vi "Load WFM Data.vi"(4 "error in (no error)":errorcluster, 5 "# Records (1)":i32=1, 6 "# Records to Skip (0)":i32, 7 "Source File":path) -> (0 "error out":errorcluster, 3 "Data":waveform(dbl)[][](array[waveform]))   [LabVIEW 2013]
panel:
  out "Records read":i32
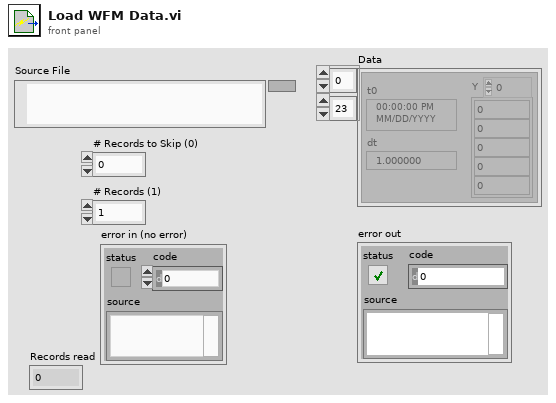
[diagram p1: front panel]
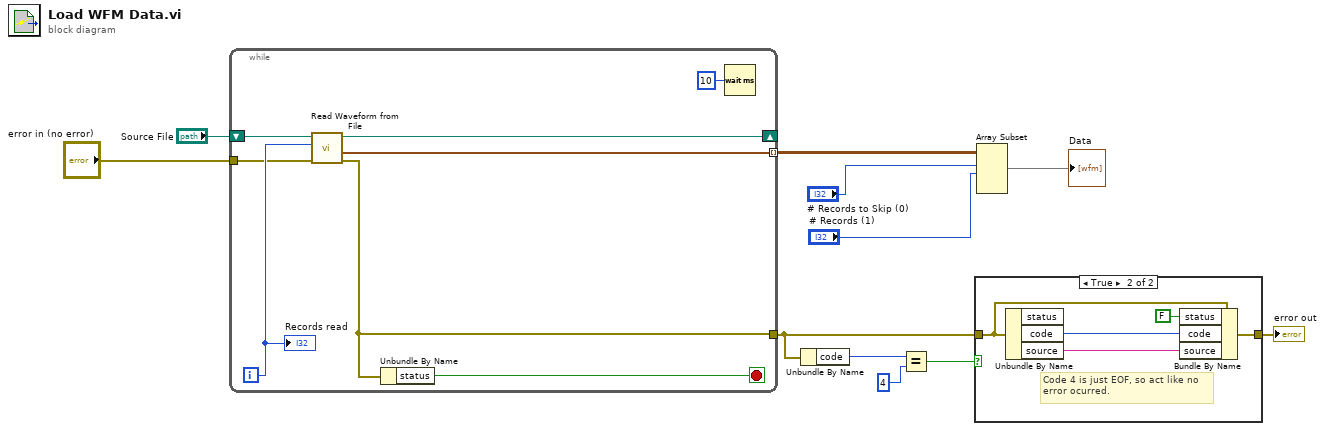
[diagram p0: block diagram]
diagram:
  n1 = while {
    tunnel: [w16] -> w7 mode=indexing
    shift-right: [w15] -> _
    shift-left: "Source File" -> [w14]
    tunnel: [w13] -> w4
    tunnel: "error in (no error)" -> [w12]
    i -> [w19]
    stop <- w18 stop-if-true
    n2 = call <vilib>:"Read Waveform from File.vi"("error in (no error)"=w12, "offset (records:0)"=w19, "file path (dialog if empty)"=w14) -> ("error out"=w13:errorcluster, "all waveforms in record"=w16:waveform(dbl)[], "new file path (Not A Path if cancelled)"=w15:path)  [unwired: 3 in, 1 out]
    n3 = Unbundle By Name(w13) -> ("status"=w18:bool)
    n4 = Wait (ms)(milliseconds to wait=u32 10) -> ()  [unwired: 1 out]
    "Records read" <- w19
  }
  n5 = Unbundle By Name(w4) -> ("code"=w3:i32)
  n6 = Equal?(x=w3, y=4 ("code")) -> (x = y?=w11:bool)
  n7 = case shown="True" w11 {
    tunnel: w4 -> [w20 w25]
    tunnel: [w20 w21] -> w9
    frame False {
    }
    frame True {
      # "Code 4 is just EOF, so act like no\nerror ocurred."
      n8 = Unbundle By Name(w25) -> ("code"=w24:i32, "source"=w23:string)  [unwired: 1 out]
      n9 = Bundle By Name(cluster=w25, "status"=FALSE, "code"=w24, "source"=w23) -> (w21:errorcluster)
    }
  }
  "error out" <- w9
  n10 = Array Subset(array=w7, index (row)="# Records to Skip (0)", length (row)="# Records (1)") -> (→"Data":waveform(dbl)[][])  [unwired: 2 in]
